vi "Shutdown App Manager.vi"(8 "error in (no error)":errorcluster, 11 "teststand-api in":refnum<class "teststand-api.lvclass">) -> (0 "error out":errorcluster, 2 "Shutdown":bool, 3 "teststand-api out":refnum<class "teststand-api.lvclass">)   [LabVIEW 2014, in "teststand-api.lvlib" / "teststand-api.lvclass"]
uses:
  teststand-api.lvclass
  teststand-api.lvclass/teststand-api.ctl
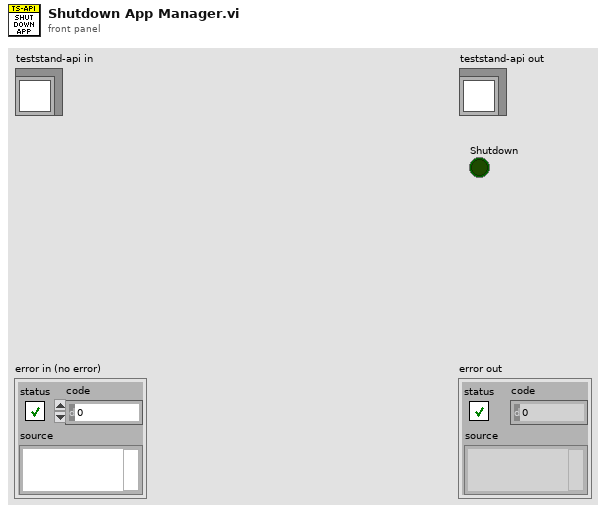
[diagram p1: front panel]
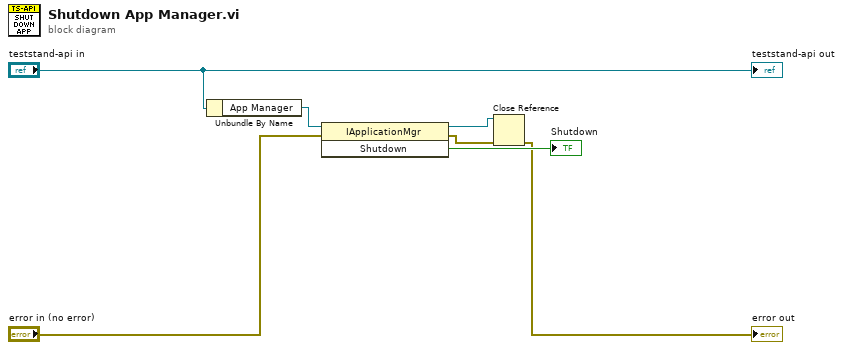
[diagram p0: block diagram]
diagram:
  n1 = Unbundle By Name("teststand-api in") -> ("App Manager"=w6:refnum<k7>)
  n2 = invoke class="IApplicationMgr" method="Shutdown"(reference=w6, error in="error in (no error)") -> (reference out=w3:refnum<k7>, error out=w2:errorcluster, "Shutdown"=→"Shutdown":bool)  [unwired: 1 in]
  n3 = Close Reference(reference=w3, error in (no error)=w2) -> (error out=→"error out":errorcluster)
  "teststand-api out" <- "teststand-api in"
